vi "LinxClose.vi"(8 "Error In":errorcluster, 11 "LINX Resource":T1) -> (0 "Error Out":errorcluster, 3 "LINX Resource":T1)   [LabVIEW 2020, in "LMH-LINX.lvlib" / "Local IO.lvlib"]
uses:
  Local IO.lvlib
  Type Defs/LINX Ref.ctl
  Type Defs/Platform.ctl
  Device/Type Defs/LINX Device Config.ctl
  Type Defs/Interface.ctl
  Device/Type Defs/TCP Config.ctl
  Device/Type Defs/Channels.ctl
  Resources/liblinxdevice.dll
  LMH-LINX.lvlib
  Device/Device.lvlib
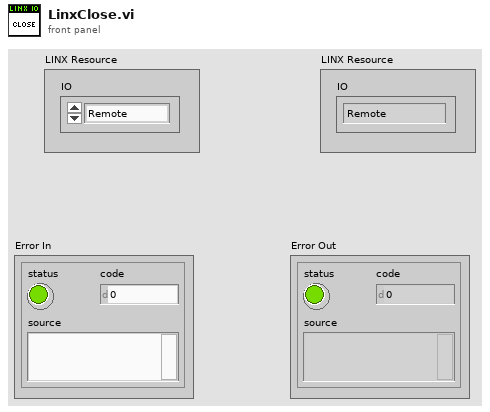
[diagram p1: front panel]
types:
  T1 = typedef "LMH-LINX.lvlib/LINX Ref.ctl" = cluster{"IO":T2, "LINX Device Config":T3}
  T2 = typedef "LMH-LINX.lvlib/Platform.ctl" = enum16{"Remote", "Local"}
  T3 = typedef "Device.lvlib/LINX Device Config.ctl" = cluster{"Interface":T4, "COM Port":refnum<visa-resource-name>, "TCP Configuration":T5, "Device Family":u8, "Device ID":u8, "Device Name":string, "TCP Ref":refnum<k5>, "Local Refnum":u64, "Channels":T6}
  T4 = typedef "LMH-LINX.lvlib/Interface.ctl" = enum16{"Serial", "TCP"}
  T5 = typedef "Device.lvlib/TCP Config.ctl" = cluster{"IP Address":string, "Port":u16}
  T6 = typedef "LMH-LINX.lvlib/Channels.ctl" = cluster{"DI":u8[], "DO":u8[], "AI":u8[], "AO":u8[], "PWM":u8[], "QE":u8[], "UART":u8[], "I2C 2":u8[], "SPI":u8[], "CAN":u8[], "Servo":u8[], "AI Ref (V)":dbl, "AI Resolution (Bits)":u8, "AO Ref (V)":dbl, "AO Resolution (Bits)":u8}
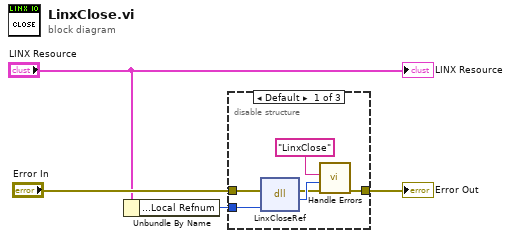
[diagram p0: block diagram]
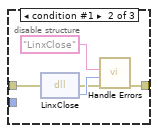
[diagram p2: hidden frame]
diagram:
  n1 = Unbundle By Name("LINX Resource") -> ("LINX Device Config.Local Refnum"=w1:u64)
  n2 = disable-structure shown="Default" {
    disable-tunnel: [w6 w12 w16] -> w3
    disable-tunnel: "Error In" -> [w7 w11 w16]
    disable-tunnel: w1 -> [w5 _ _]
    frame condition #0 (active) {
      n3 = dll-call lib="C:/Users/rkalbermatter/Projects/LabVIEW Hobbyist/LabVIEW/vi.lib/MakerHub/LINX/Resources/liblinxdevice.*" fn="LinxCloseRef"(error in=w7, "refnum"=w5) -> (error out=w9:errorcluster, "LinxStatus"=w10:i32)  [unwired: 3 in, 1 out]
      n4 = call "Handle Errors.vi"("Error In"=w9, "LinxStatus"=w10, "Function Name"="LinxClose") -> ("Error Out"=w6:errorcluster)  [unwired: 7 in, 1 out]
    }
    frame condition #1 {
      n5 = dll-call lib="C:/Users/rkalbermatter/Projects/LabVIEW Hobbyist/LabVIEW/vi.lib/MakerHub/LINX/Resources/liblinxdevice.*" fn="LinxClose"(error in=w11) -> (error out=w13:errorcluster, "LinxStatus"=w14:i32)  [unwired: 2 in, 1 out]
      n6 = call "Handle Errors.vi"("Error In"=w13, "LinxStatus"=w14, "Function Name"="LinxClose") -> ("Error Out"=w12:errorcluster)  [unwired: 7 in, 1 out]
    }
    frame condition #2 {
      # "1900 | 1950"
    }
  }
  "Error Out" <- w3
  "LINX Resource" <- "LINX Resource"
